vi "FromRepo.vi"(8 "error in":errorcluster, 9 "cluster":T2, 10 "repository in":refnum<class "NISE_CEF_Repository.lvclass">, 11 "CleanupCategoryNode in":refnum<class "CleanupCategoryNode.lvclass">) -> (0 "error out":errorcluster, 2 "repository out":refnum<class "NISE_CEF_Repository.lvclass">, 3 "node":T1)   [LabVIEW 2015, in "CleanupCategoryNode.lvclass"]
doc: "Copyright 2017 National Instruments Corporation\n\nLicensed under the Apache License, Version 2.0 (the \"License\"); you may not use this file except in compliance with the License. You may obtain a copy of the License at http://www.apache.org/licenses/LICENSE-2.0\nUnless required by applicable law or agreed to in writing, software distributed under the License is distributed on an \"AS IS\" BASIS, WITHOUT WARRANTIES OR CONDITIONS OF ANY KIND, either express or implied. See the License for the specific language governing permissions and limitations under the License."
uses:
  CleanupCategoryNode.lvclass
  <vilib>/NI/Configuration Framework/Repository/NISE_CEF_Repository.lvclass
  <vilib>/NI/Configuration Framework/Node/FromRepoCluster.ctl
  <vilib>/NI/Configuration Framework/Node/NodeRef.ctl
  <vilib>/NI/Configuration Framework/Node/NISE_CEF_Node.lvclass
  SequenceRepo/SequenceRepo.lvclass
  Prototype/classes/Sequence/Config/Sequence Config.lvclass
  Prototype/classes/Step/Config/Step Config.lvclass
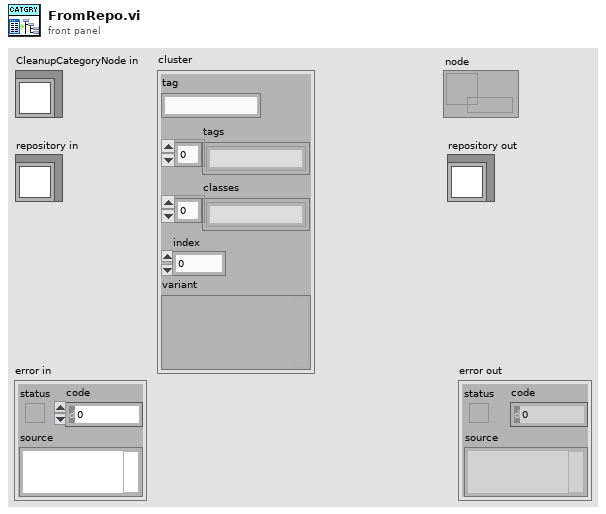
[diagram p1: front panel]
types:
  T1 = typedef "NISE_CEF_Node.lvclass/NodeRef.ctl" = refnum<data-value>
  T2 = typedef "NISE_CEF_Node.lvclass/FromRepoCluster.ctl" = cluster{"tag":string, "tags":string[], "classes":string[], "index":i32, "variant":variant}
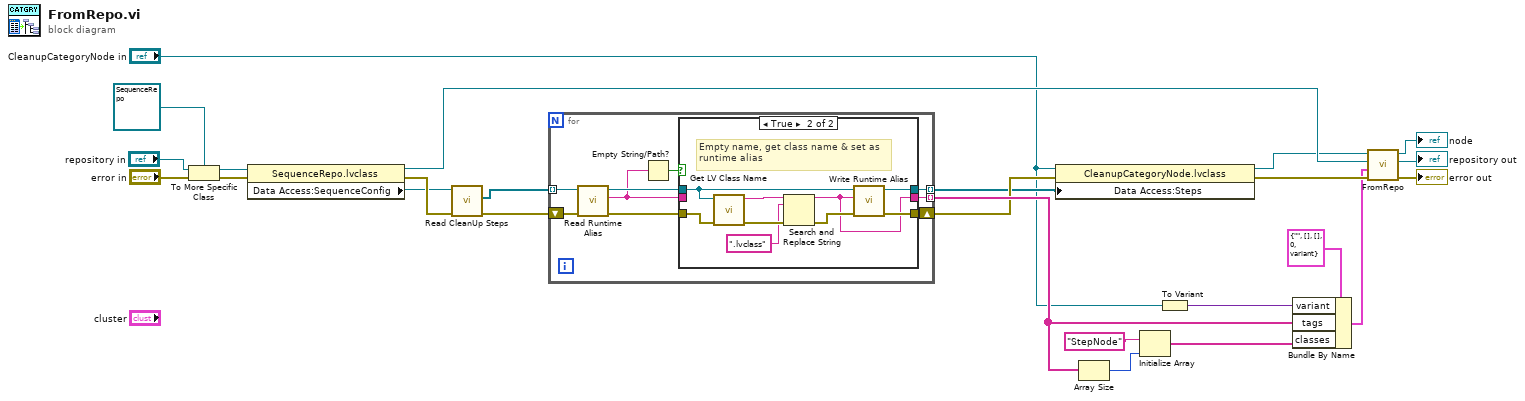
[diagram p0: block diagram]
diagram:
  n1 = To More Specific Class(target class=refnum<class "SequenceRepo.lvclass"> refnum ("cRIO repo.lvclass"), reference="repository in", error in="error in") -> (specific class reference=w21:refnum<class "SequenceRepo.lvclass">, error out=w18:errorcluster)
  n2 = property class="SequenceRepo.lvclass"(reference=w21, error in=w18) -> (reference out=w20:refnum<class "SequenceRepo.lvclass">, error out=w15:errorcluster, "Data Access:SequenceConfig"=w14:refnum<class "Sequence Config.lvclass">)
  n3 = call-dynamic "Read CleanUp Steps .vi"("error in (no error)"=w15, "Sequence Config in"=w14) -> ("error out"=w8:errorcluster, "CleanUp Steps"=w6:refnum<class "Step Config.lvclass">[])  [unwired: 7 in, 1 out]
  n4 = for {
    tunnel: [w26] -> w9 mode=indexing
    shift-right: [w31] -> w7
    shift-left: w8 -> [w34]
    tunnel: w6 -> [w32] mode=indexing
    tunnel: [w27] -> w3 mode=indexing
    n5 = call-dynamic "Read Runtime Alias.vi"("error in (no error)"=w34, "Step Config in"=w32) -> ("error out"=w33:errorcluster, "Runtime Alias"=w28:string, "Step Config out"=w30:refnum<class "Step Config.lvclass">)  [unwired: 7 in]
    n6 = Empty String/Path?(string/path=w28) -> (empty?=w29:bool)
    n7 = case shown="True" w29 {
      tunnel: w33 -> [w37 w46]
      tunnel: [w37 w41] -> w31
      tunnel: w30 -> [w36 w40]
      tunnel: w28 -> [w35 _]
      tunnel: [w36 w39] -> w27
      tunnel: [w35 w38] -> w26
      frame False {
        # "runtime alias already exists, use"
      }
      frame True {
        # "Empty name, get class name & set as runtime alias"
        n8 = call <vilib>:"Get LV Class Name.vi"("error in (no error)"=w46, "object"=w40) -> ("error out"=w44:errorcluster, "class name"=w45:string)  [unwired: 8 in]
        n9 = Search and Replace String(input string=w45, search string=".lvclass", error in=w44) -> (result string=w38:string, error out=w43:errorcluster)  [unwired: 5 in, 2 out]
        n10 = call-dynamic "Write Runtime Alias.vi"("error in (no error)"=w43, "Runtime Alias"=w38, "Step Config in"=w40) -> ("error out"=w41:errorcluster, "Step Config out"=w39:refnum<class "Step Config.lvclass">)  [unwired: 7 in]
      }
    }
  }
  n11 = property class="CleanupCategoryNode.lvclass"(reference="CleanupCategoryNode in", error in=w7, "Data Access:Steps"=w3) -> (reference out=w4:refnum<class "CleanupCategoryNode.lvclass">, error out=w17:errorcluster)
  n12 = Array Size(array=w9) -> (size(s)=w12:i32)
  n13 = Initialize Array("StepNode" ("System"), w12) -> (w10:string[])
  n14 = To Variant(anything="CleanupCategoryNode in") -> (Variant=w1:variant)
  n15 = Bundle By Name(cluster=T2 {"tag"="", "tags"=[], "classes"=[], "index"=0, "variant"=variant} ("Cluster"), "variant"=w1, "tags"=w9, "classes"=w10) -> (w5:T2)
  n16 = call-parent "FromRepo.vi"("error in"=w17, "from repo cluster"=w5, "repository in"=w20, "node in"=w4) -> ("error out"=→"error out":errorcluster, "repository out"=→"repository out":refnum<class "NISE_CEF_Repository.lvclass">, "node"=→"node":T1)  [unwired: 5 in]
